vi "ITISignal.vi"(1 "SL":dbl, 2 "NV":dbl) -> (0 "Logging":dbl(graph))   [LabVIEW 2014]
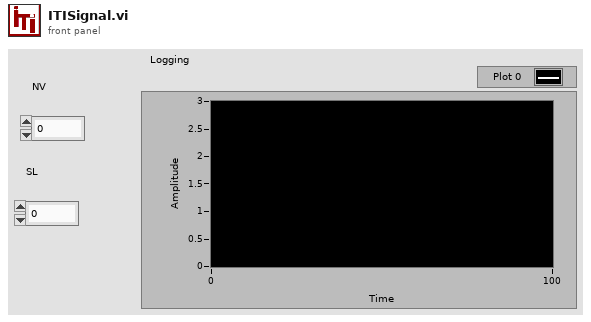
[diagram p1: front panel]
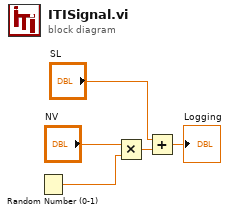
[diagram p0: block diagram]
diagram:
  n1 = Random Number (0-1)() -> (number: 0 to 1=w5:dbl)
  n2 = Multiply(x="NV", y=w5) -> (x*y=w3:dbl)
  n3 = Add(x="SL", y=w3) -> (x+y=→"Logging":dbl)
